vi "Camera-SetUp-Acquisition.vi"(9 "Laser Shutter":T1=enum."Off", 10 "Image Size":T4={"H Bin"=1.0, "V Bin"=1.0, "Left"=1.0, "Right"=1024.0, "Top"=1.0, "Bottom"=1024.0} {"V Bin" min=0.0; "H Bin" min=0.0 step=1.0}, 11 "Acquisition Parameters":T5={"Readout Mode"=enum."Image", "Set Acquisition Mode"=enum."Single Scan", "Trigger Mode"=enum."Internal", "Exposure Time (sec)"=1.0, "Accumulation Cycle (s)"=1.0, "Kinetic Cycle Time (s)"=1.0, "Number of Kinetics"=1, "Number of Accumulations"=1, "Set VS Speed"=1.0, "Pixel Rate"=enum."Standard CCD 3 Mhz 14 bits", "V Shift Amplitude"=enum."+1", "Preamp Gain"=enum."1.0", "Single Track Settings"={"centre"=0, "height"=1}, "EM CCD Gain"=300, "High Capacity?"=FALSE} {"EM CCD Gain" scale=0.01..300.0; "Single Track Settings"."centre" min=0 max=1024; "Single Track Settings"."height" min=1 max=1024; "Exposure Time (sec)" scale=0.001..10.0 scale format="%#_1g"; "Set VS Speed" min=0.0 format="%#_2f"}) -> (0 "Error Out":errorcluster, 1 "File properties":T2, 2 "Image Size Out":T3 {"V Bin" min=0.0; "H Bin" min=0.0 step=1.0}, 3 "Continue with acq?":bool)   [LabVIEW 2014]
uses:
  SubVIs/ctt's/Camera Setup Acquisition.ctl
  SubVIs/ctt's/Image size and binning.ctl
  SubVIs/ctt's/acquisition control.ctl
  Shutter Control/Shutter SubVIs/ctts/laser shutters.ctl
  SubVIs/ctt's/image-acquision 2.ctl
  <vilib>/vision/Image Controls.llb/IMAQ Image.ctl
  Shutter Control/Shutter SubVIs/ctts/control shutters.ctl
  SubVIs/Globals/Initilize Globals.vi
  TIRF Lock/autofocus-globals.vi
panel:
  in  "Display Live\nvideo":bool
  in  "Continous autofocus\nduring preview?":bool
  out "Actual Exposure Time (sec)":dbl
  in  "STOP":bool
  in  "Preview":bool
  in  "Go":bool
  in  "Number of \npreview windows":i32=1
  in  "Set to AOI":bool
  in  "Set to 512 x 300":bool
  in  "Set to Maximum":bool
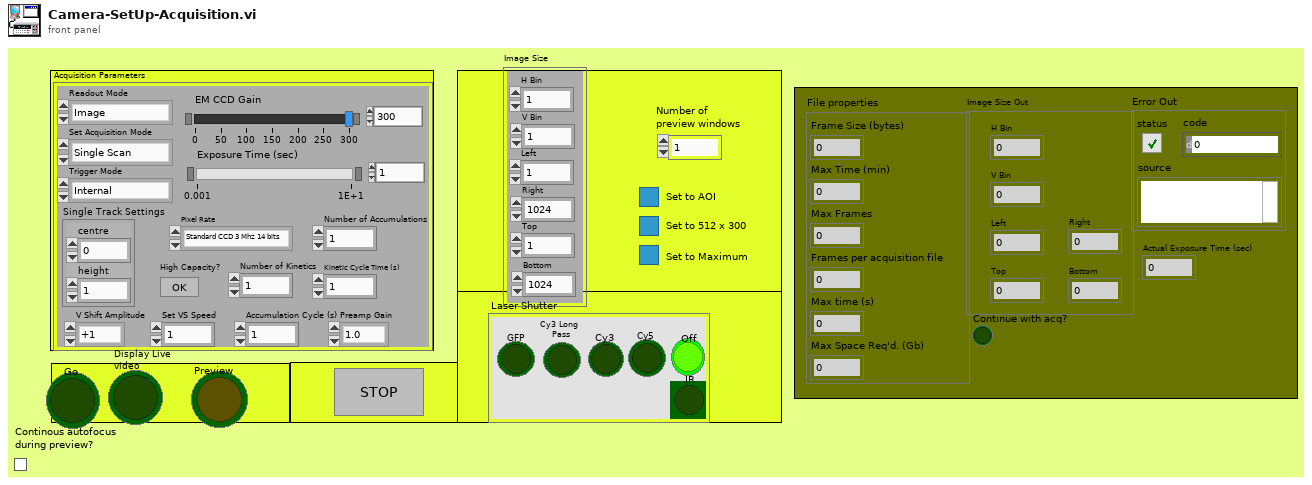
[diagram p1: front panel]
types:
  T1 = typedef "laser shutters.ctl" = enum32{"No Selection", "GFP", "Cy3 Long \nPass", "Cy3", "Cy5", "Off", "IR"}
  T2 = cluster{"Frame Size (bytes)":i32, "Max Time (min)":i32, "Max Frames":i32, "Frames per acquisition file":i32, "Max time (s)":i32, "Max Space Req'd. (Gb)":dbl}
  T3 = typedef "acquisition control.ctl" = cluster{"H Bin":dbl, "V Bin":dbl, "Left":dbl, "Right":dbl, "Top":dbl, "Bottom":dbl}
  T4 = typedef "Image size and binning.ctl" = cluster{"H Bin":dbl, "V Bin":dbl, "Left":dbl, "Right":dbl, "Top":dbl, "Bottom":dbl}
  T5 = typedef "Camera Setup Acquisition.ctl" = cluster{"Readout Mode":enum16{"Full Vertical Binning", "Multi-Track", "Random-Track", "Single-Track", "Image"}, "Set Acquisition Mode":enum16{"(do nothing)", "Single Scan", "Accumulate", "Kinetics", "Fast Kinetics", "Run till abort"}, "Trigger Mode":enum16{"Internal", "External"}, "Exposure Time (sec)":sgl, "Accumulation Cycle (s)":dbl, "Kinetic Cycle Time (s)":dbl, "Number of Kinetics":i32, "Number of Accumulations":i32, "Set VS Speed":dbl, "Pixel Rate":enum16{"EM CCD 10 Mhz 14 bits", "EM CCD 5 Mhz 14 bits", "EM CCD 3 Mhz 14 bits", "EM CCD 1 Mhz 16 bits", "Standard CCD 3 Mhz 14 bits", "Standard CCD 1 Mhz 16 bits"}, "V Shift Amplitude":enum16{"normal", "+1", "+2", "+3", "+4"}, "Preamp Gain":enum16{"1.0", "2.4", "5.0"}, "Single Track Settings":cluster{"centre":i32, "height":i32}, "EM CCD Gain":u16, "High Capacity?":bool}
  T6 = typedef "image-acquision 2.ctl" = u32
  T7 = typedef "IMAQ Image.ctl" = refnum<image>
  T8 = typedef "control shutters.ctl" = cluster{"Camera Shutter":bool, "Laser Shutter":enum32{"No Selection", "GFP", "Cy3 Long \nPass", "Cy3", "Cy5", "Off"}}
  T9 = cluster{"H Bin":dbl, "V Bin":dbl, "Left":dbl, "Right":dbl, "Top":dbl, "Bottom":dbl}
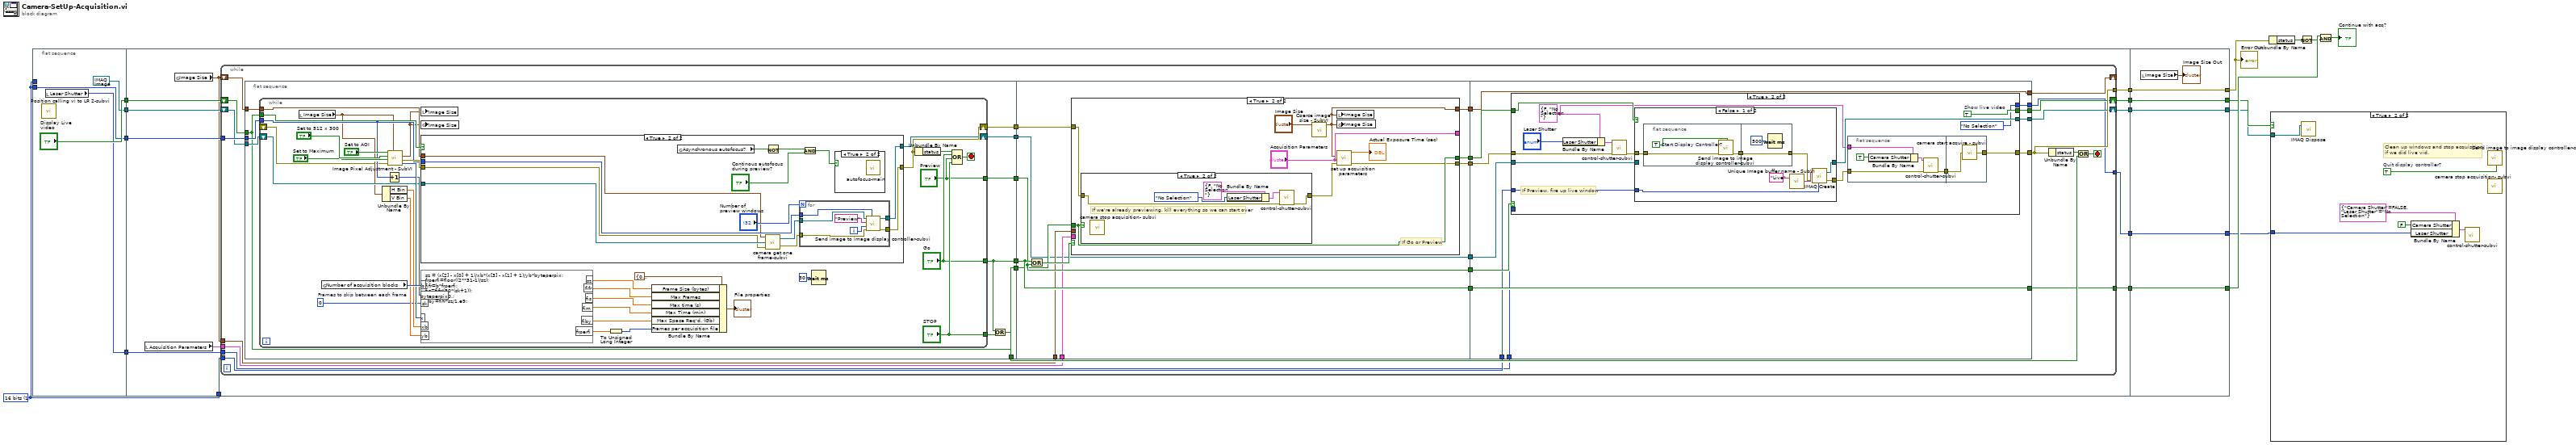
[diagram p0: block diagram]
diagram:
  w3 = T6 1 items=["8 bits", "16 bits", "Float", "Complex", "RGB", "HSL"] ("Image Type")
  n1 = flat-sequence {
    tunnel: ["Display Live\nvideo"] -> w18
    tunnel: [w21] -> w17
    tunnel: w3 -> [w21]
    tunnel: [T7 refnum ("Image")] -> w16
    tunnel: [w19] -> w15
    tunnel: w3 -> [_]
    tunnel: w18 -> [w34]
    tunnel: w17 -> [w33]
    tunnel: w16 -> [w32]
    tunnel: w15 -> [w30]
    tunnel: w3 -> [w31]
    tunnel: [w29] -> w14
    tunnel: [w28] -> w13
    tunnel: [w27] -> w12
    tunnel: [w26] -> w11
    tunnel: [w23] -> w2
    tunnel: [w215] -> w4
    tunnel: w14 -> [w215]
    tunnel: [w214] -> w6
    tunnel: w13 -> [w214]
    tunnel: [w213] -> w5
    tunnel: w12 -> [w213]
    tunnel: [w212] -> w10
    tunnel: w11 -> [w212]
    tunnel: [w210] -> w1
    tunnel: w2 -> [w210]
    frame #0 {
      n2 = call "Position calling vi to LR 2-subvi.vi"() -> ()  [unwired: 4 in, 2 out]
      n3 = local read "Laser Shutter"() -> (w19:T1)
    }
    frame #1 {
      n4 = local read "Acquisition Parameters"() -> (w24:T5)
      n5 = global read "Initilize Globals.vi" "Image Size"() -> (w25:T4)
      n6 = while {
        shift-right: [w40] -> w28
        shift-left: w34 -> [w62]
        tunnel: w33 -> [w61]
        shift-right: [w39] -> w27
        shift-left: w32 -> [w60]
        shift-right: [w38] -> _
        shift-left: w25 -> [w59]
        tunnel: w25 -> [w49]
        tunnel: w24 -> [w48]
        tunnel: w31 -> [w43]
        tunnel: w30 -> [w42]
        tunnel: [w36] -> w26
        tunnel: [w35] -> w23
        tunnel: [w41] -> w29
        stop <- w56 stop-if-true
        n7 = flat-sequence {
          tunnel: w62 -> [w64]
          tunnel: w61 -> [w72]
          tunnel: w60 -> [w71]
          tunnel: w59 -> [w70]
          tunnel: [w68] -> w58
          tunnel: [w67] -> w57
          tunnel: [w66] -> w55
          tunnel: [w65] -> w53
          tunnel: [w64] -> w52
          tunnel: [w63] -> w47
          tunnel: w58 -> [w138]
          tunnel: w57 -> [w139]
          tunnel: w53 -> [w133]
          tunnel: w52 -> [w136]
          tunnel: [w139] -> w51
          tunnel: [w138] -> w50
          tunnel: w49 -> [w135]
          tunnel: w48 -> [w134]
          tunnel: w47 -> [w132]
          tunnel: [w132] -> w46
          tunnel: [w131] -> w45
          tunnel: [w130] -> w44
          tunnel: [w129] -> w37
          tunnel: w51 -> [w168]
          tunnel: w50 -> [w169]
          tunnel: w46 -> [w167]
          tunnel: [w168] -> w36
          tunnel: w45 -> [w166]
          tunnel: w44 -> [w165]
          tunnel: w43 -> [w164]
          tunnel: w42 -> [w163]
          tunnel: [w162] -> w41
          tunnel: [w161] -> w40
          tunnel: [w160] -> w39
          tunnel: [w159] -> w35
          tunnel: [w158] -> w38
          tunnel: w37 -> [w158]
          frame #0 {
            n8 = while {
              shift-right: [w84] -> w65
              shift-left: _ -> [w73]
              tunnel: w64 -> [w89]
              tunnel: w72 -> [w85]
              shift-right: [w83] -> w63
              shift-left: w71 -> [w88]
              tunnel: w70 -> [w87]
              tunnel: ["STOP"] -> w69
              tunnel: ["Go"] -> w67
              tunnel: ["Preview"] -> w68
              stop <- w81 stop-if-true
              w98 = u16 0  # Frames to skip between each frame
              n9 = local read "Image Size"() -> (w75:T4)
              n10 = global read "Initilize Globals.vi" "Number of acquisition blocks"() -> (w102:i8)
              n11 = Unbundle By Name(w75) -> ("H Bin"=w100:dbl, "V Bin"=w99:dbl)
              n12 = Increment(x=w85) -> (x+1=w97:T6)
              n13 = call "Image Pixel Adjustment - SubVI.vi"("Image Size"=w75, "error in"=w73, "Set to Maximum"="Set to Maximum", "Set to 512 x 300"="Set to 512 x 300", "Set to AOI"="Set to AOI") -> ("Pixels Out"=w101:i32[], "Error Out (no error)"=w86:errorcluster, "Image Size 2"=w74:T9)  [unwired: 4 in]
              n14 = local write "Image Size"(w74) -> ()
              n15 = global write "Initilize Globals.vi" "Image Size"(w74) -> ()
              n16 = case shown="True" w89 {
                tunnel: w88 -> [w108 w121]
                tunnel: [w108 w115] -> w83
                tunnel: w87 -> [_ w113]
                tunnel: w86 -> [w107 w120]
                tunnel: w85 -> [_ w116]
                tunnel: [w107 w114] -> w84
                frame False {
                }
                frame True {
                  n17 = global read "autofocus-globals.vi" "Asynchronous autofocus?"() -> (w109:bool)
                  n18 = call "camera get one frame-subvi.vi"("error in"=w120, "New Image"=w121, "Image Size"=w113) -> ("error out"=w117:errorcluster, "Image Out"=w118:T7)
                  n19 = Not(x=w109) -> (.not. x?=w110:bool)
                  n20 = for {
                    N: "Number of \npreview windows" -> [_]
                    tunnel: w118 -> [w126]
                    tunnel: w117 -> [w127]
                    tunnel: w116 -> [w128]
                    tunnel: [w123] -> w115
                    tunnel: [w122] -> w114
                    i -> [w124]
                    n21 = call "Send image to image display controller-subvi.vi"("Image"=w126, "Window Title"="Preview" ("Window Title\n(Window only)"), "Window Number"=w124, "error in"=w127, "Image Type"=w128) -> ("Image Out"=w123:T7, "error out"=w122:errorcluster)  [unwired: 4 in]
                  }
                  n22 = And(x=w110, y="Continous autofocus\nduring preview?") -> (x .and. y?=w112:bool)
                  n23 = case shown="True" w112 {
                    frame False {
                    }
                    frame True {
                      n24 = call "autofocus-main.vi"() -> ()  [unwired: 12 in]
                    }
                  }
                }
              }
              n25 = formula code="sz = (x[2] - x[0] + 1)/xb*(x[3] - x[1] + 1)/yb*byteperpix;\nfrperfi=floor((2**31-1)/sz);\nfifr=b*frperfi;\nfis=fifr/(30*(sk+1));\nfim=fis/60.;\nfiby=fifr*sz/1.e9;"("x"=w101, "b"=w102, "sk"=w98, "xb"=w100, "yb"=w99, "byteperpix"=w97) -> ("sz"=w90:dbl, "fifr"=w91:dbl, "fis"=w92:dbl, "fim"=w93:dbl, "fiby"=w94:dbl, "frperfi"=w96:dbl)
              n26 = To Unsigned Long Integer(number=w96) -> (unsigned 32bit integer=w95:u32)
              n27 = Bundle By Name(cluster=T2 {"Frame Size (bytes)"=0, "Max Time (min)"=0, "Max Frames"=0, "Frames per acquisition file"=0, "Max time (s)"=0, "Max Space Req'd. (Gb)"=0.0}, "Frame Size (bytes)"=w90, "Max Frames"=w91, "Max time (s)"=w92, "Max Time (min)"=w93, "Max Space Req'd. (Gb)"=w94, "Frames per acquisition file"=w95) -> (→"File properties":T2)
              n28 = Wait (ms)(milliseconds to wait=u32 30) -> ()  [unwired: 1 out]
              n29 = Unbundle By Name(w84) -> ("status"=w82:bool)
              n30 = Compound Arithmetic op=OR(w82, "Go", "Preview", "STOP") -> (w81:bool)
            }
            n31 = Or(x=w67, y=w69) -> (x .or. y?=w66:bool)
          }
          frame #1 {
            n32 = Or(x=w139, y=w138) -> (x .or. y?=w137:bool)
            n33 = case shown="True" w137 {
              tunnel: w136 -> [w143 w151]
              tunnel: [w143 w151] -> w130
              tunnel: [w141 "Acquisition Parameters"] -> _
              tunnel: [w142 w144] -> w129
              tunnel: w135 -> [w142 _]
              tunnel: w134 -> [w141 _]
              tunnel: w133 -> [w140 w148]
              tunnel: [w140 w145] -> w131
              frame False {
              }
              frame True {
                # "If Go or Preview"
                n34 = case shown="True" w151 {
                  tunnel: w148 -> [w152 w155]
                  tunnel: [w152 w154] -> w147
                  frame False {
                  }
                  frame True {
                    # "If we're already previewing, kill everything so we can start over"
                    n35 = call "camera stop acquisition- subvi.vi"() -> ()  [unwired: 1 in]
                    n36 = Bundle By Name(cluster=T8 {"Camera Shutter"=FALSE, "Laser Shutter"=enum."No Selection"} ("Shutter Control"), "Laser Shutter"=laser_shutters."No Selection" ("Laser Shutter 2")) -> (w153:T8)
                    n37 = call "control-shutter-subvi.vi"("Error In"=w155, "Shutter Control"=w153) -> ("Error Out"=w154:errorcluster)  [unwired: 9 in]
                  }
                }
                n38 = call "Coerce image size - SubVI.vi"("Image Size"="Image Size") -> ("Image Size 2"=w144:T9)  [unwired: 10 in]
                n39 = local write "Image Size"(w144) -> ()
                n40 = global write "Initilize Globals.vi" "Image Size"(w144) -> ()
                n41 = call "set up acquisition parameters.vi"("error in (no error)"=w147, "Acquisition Parameters"="Acquisition Parameters", "Image Size"=w144) -> ("error out"=w145:errorcluster, "Exposure (s)"=→"Actual Exposure Time (sec)":dbl)  [unwired: 3 in, 2 out]
              }
            }
          }
          frame #2 {
            n42 = case shown="True" w169 {
              tunnel: w167 -> [w170 w186]
              tunnel: w166 -> [w173 w178]
              tunnel: w165 -> [w171 w187]
              tunnel: [w173 w181] -> w162
              tunnel: w164 -> [_ w185]
              tunnel: [w171 w184] -> w161
              tunnel: [w172 laser_shutters."No Selection" ("Laser Shutter")] -> w159
              tunnel: w163 -> [w172 _]
              tunnel: [w170 w180] -> w160
              frame False {
              }
              frame True {
                w176 = T8 {"Camera Shutter"=FALSE, "Laser Shutter"=enum."No Selection"} ("Shutter Control")
                w184 = TRUE  # Show live video
                # "If Preview, fire up live window"
                n43 = Bundle By Name(cluster=w176, "Laser Shutter"="Laser Shutter") -> (w179:T8)
                n44 = call "control-shutter-subvi.vi"("Error In"=w178, "Shutter Control"=w179) -> ("Error Out"=w177:errorcluster)  [unwired: 9 in]
                n45 = case shown="False" w187 {
                  tunnel: w177 -> [w202 w208]
                  tunnel: w186 -> [_ w209]
                  tunnel: [w199 w209] -> w180
                  tunnel: [w200 w208] -> w183
                  tunnel: w185 -> [w196 _]
                  frame False {
                    n46 = flat-sequence {
                      tunnel: w202 -> [w205]
                      tunnel: [w203] -> w201
                      tunnel: [w207] -> w195
                      tunnel: w201 -> [w207]
                      frame #0 {
                        w204 = TRUE  # Start Display Controller?
                        n47 = call "Send image to image display controller-subvi.vi"("error in"=w205, "Start display controller?"=w204) -> ("error out"=w203:errorcluster)  [unwired: 7 in, 1 out]
                      }
                      frame #1 {
                        n48 = Wait (ms)(milliseconds to wait=u32 500) -> ()  [unwired: 1 out]
                      }
                    }
                    n49 = call "Unique Image buffer name - SubVI.vi"("Buffer  base name"="Live") -> ("Image Name"=w198:string)  [unwired: 1 in]
                    n50 = call "IMAQ Create"("Image Name"=w198, "Image Type"=w196, "error in (no error)"=w195) -> ("New Image"=w199:T7, "error out"=w200:errorcluster)  [unwired: 1 in, 1 out]
                  }
                  frame True {
                  }
                }
                n51 = flat-sequence {
                  tunnel: w183 -> [w191]
                  tunnel: [w192] -> w182
                  tunnel: w176 -> [w190]
                  tunnel: w182 -> [w194]
                  tunnel: [w193] -> w181
                  frame #0 {
                    n52 = Bundle By Name(cluster=w190, "Camera Shutter"=TRUE) -> (w188:T8)
                    n53 = call "control-shutter-subvi.vi"("Error In"=w191, "Shutter Control"=w188) -> ("Error Out"=w192:errorcluster)  [unwired: 9 in]
                  }
                  frame #1 {
                    n54 = call "camera start acquire - subvi.vi"("error in"=w194) -> ("error out"=w193:errorcluster)
                  }
                }
              }
            }
          }
        }
        n55 = Unbundle By Name(w41) -> ("status"=w54:bool)
        n56 = Or(x=w54, y=w55) -> (x .or. y?=w56:bool)
      }
    }
    frame #2 {
      n57 = local read "Image Size"() -> (→"Image Size Out":T4)
    }
  }
  n58 = Unbundle By Name(w4) -> ("status"=w9:bool)
  n59 = case shown="True" w6 {
    tunnel: w5 -> [_ w220]
    tunnel: w1 -> [_ w217]
    frame False {
    }
    frame True {
      w221 = TRUE  # Quit display controller?
      # "Clean up windows and stop acquisition\nif we did live vid."
      n60 = call "IMAQ Dispose"("Image"=w220) -> ()  [unwired: 2 in, 4 out]
      n61 = Bundle By Name(cluster=T8 {"Camera Shutter"=FALSE, "Laser Shutter"=enum."No Selection"} ("Shutter Control"), "Camera Shutter"=FALSE, "Laser Shutter"=w217) -> (w218:T8)
      n62 = call "control-shutter-subvi.vi"("Shutter Control"=w218) -> ()  [unwired: 10 in, 1 out]
      n63 = call "Send image to image display controller-subvi.vi"("Quit display controller?"=w221) -> ()  [unwired: 8 in, 2 out]
      n64 = call "camera stop acquisition- subvi.vi"() -> ()  [unwired: 1 in]
    }
  }
  n65 = Not(x=w9) -> (.not. x?=w8:bool)
  n66 = And(x=w10, y=w8) -> (x .and. y?=→"Continue with acq?":bool)
  "Error Out" <- w4
